vi "题目5.vi"() -> ()   [LabVIEW 2017]
panel:
  out "显示面板":T1 {"油量" scale=0.0..200.0; "速度（km/h）" scale=0.0..300.0; "转速（r/s）" scale=0.0..8000.0}
  out "油量指示灯":bool=TRUE
  in  "停止":bool
  in  "控制面板":T2 {"档位" scale=0.0..6.0; "油门" scale=0.0..10.0}
  out "时间":dbl
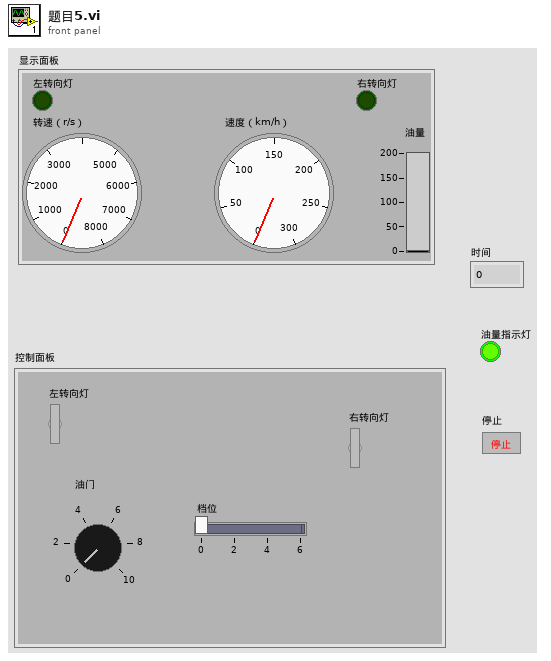
[diagram p1: front panel]
types:
  T1 = cluster{"左转向灯":bool, "右转向灯":bool, "转速（r/s）":dbl, "速度（km/h）":dbl, "油量":dbl}
  T2 = cluster{"油门":dbl, "档位":dbl, "左转向灯":bool, "右转向灯":bool}
  T3 = cluster{"左转向灯":bool, "右转向灯":bool, dbl, dbl, "y":dbl}
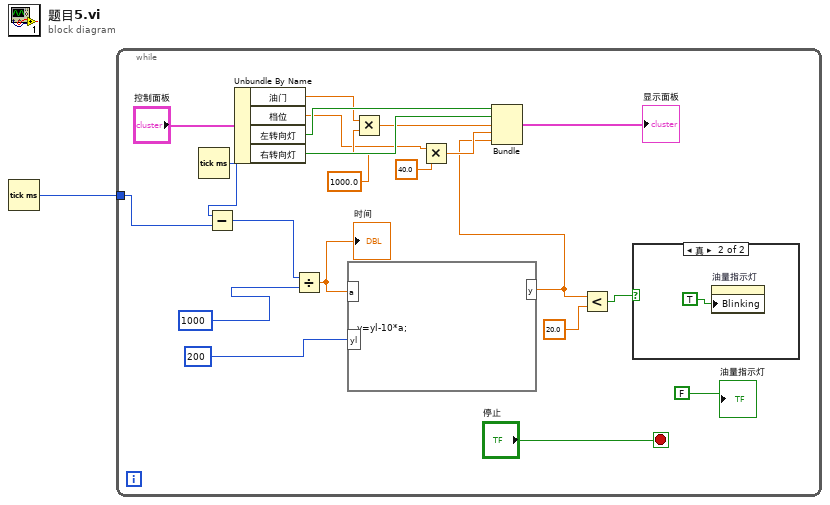
[diagram p0: block diagram]
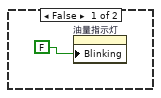
[diagram p2: hidden frame]
diagram:
  n1 = Tick Count (ms)() -> (millisecond timer value=w1:u32)
  n2 = while {
    tunnel: w1 -> [w2]
    stop <- "停止" stop-if-true
    n3 = Tick Count (ms)() -> (millisecond timer value=w22:u32)
    n4 = Subtract(x=w22, y=w2) -> (x-y=w10:u32)
    n5 = Unbundle By Name("控制面板") -> ("油门"=w18:dbl, "档位"=w14:dbl, "左转向灯"=w20:bool, "右转向灯"=w19:bool)
    n6 = Divide(x=w10, y=1000) -> (x/y=w12:dbl)
    "时间" <- w12
    n7 = formula code="y=yl-10*a;"("a"=w12, "yl"=200) -> ("y"=w8:dbl)
    n8 = Multiply(x=w18, y=1000.0) -> (x*y=w16:dbl)
    n9 = Multiply(x=w14, y=40.0) -> (x*y=w13:dbl)
    n10 = Bundle("左转向灯"=w20, "右转向灯"=w19, w16, w13, "y"=w8) -> (→"显示面板":T3)  [unwired: 1 in]
    n11 = Less?(x=w8, y=20.0) -> (x < y?=w3:bool)
    n12 = case shown="真" w3 {
      frame False {
        n13 = property on="油量指示灯" class="Bool (严格)"("Blinking"=FALSE) -> ()  [unwired: 2 in, 2 out]
      }
      frame True {
        n14 = property on="油量指示灯" class="Bool (严格)"("Blinking"=TRUE) -> ()  [unwired: 2 in, 2 out]
      }
    }
    "油量指示灯" <- FALSE
  }
